vi "INIT_temp.vi"(8 "error in (no error)":errorcluster, 11 "DelayLineLS4 in":refnum<class "DelayLineLS4.lvclass">) -> (0 "error out":errorcluster, 3 "DelayLineLS4 out":refnum<class "DelayLineLS4.lvclass">)   [LabVIEW 2015, in "DelayLineLS4.lvclass"]
uses:
  DelayLineLS4.lvclass
  DelayLine.lvclass/DelayLine.ctl
  DelayLine.lvclass
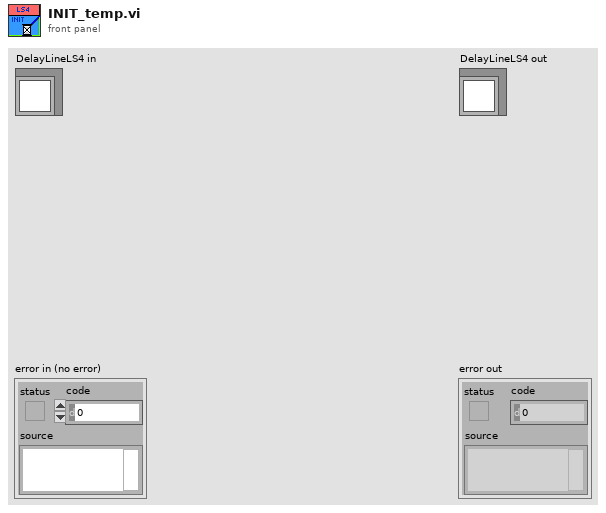
[diagram p1: front panel]
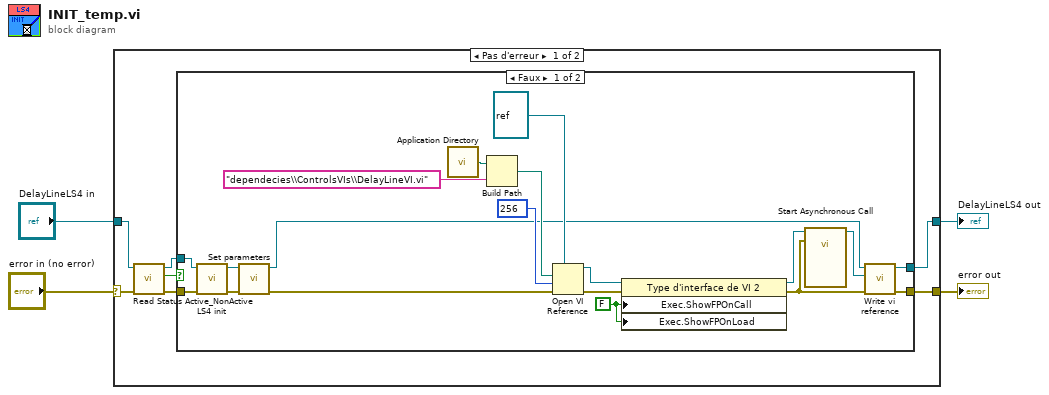
[diagram p0: block diagram]
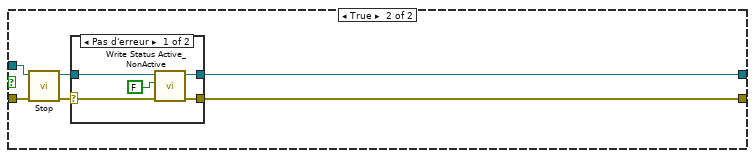
[diagram p2: hidden frame]
diagram:
  n1 = case shown="Pas d'erreur" "error in (no error)" {
    selector: "error in (no error)" -> [w8 w44]
    tunnel: "DelayLineLS4 in" -> [w7 w45]
    tunnel: [w6 w45] -> w1
    tunnel: [w5 w44] -> w2
    frame No Error {
      n2 = call "Read Status Active_NonActive.vi"("error in (no error)"=w8, "DelayLine in"=w7) -> ("error out"=w10:errorcluster, "Status Active/NonActive"=w9:bool, "DelayLine out"=w11:refnum<class "DelayLineLS4.lvclass">)  [unwired: 7 in]
      n3 = case shown="Faux" w9 {
        tunnel: w10 -> [w26 w33]
        tunnel: w11 -> [w27 w34]
        tunnel: [w30 w35] -> w5
        tunnel: [w29 w36] -> w6
        frame False {
          w15 = FALSE ("Execution:Show Front Panel On Call")
          n4 = call-dynamic "LS4 init.vi"("error in (no error)"=w26, "DelayLineLS4 in"=w27) -> ("error out"=w28:errorcluster, "DelayLineLS4 out"=w12:refnum<class "DelayLineLS4.lvclass">)  [unwired: 8 in]
          n5 = call-dynamic "Set parameters.vi"("error in (no error)"=w28, "DelayLineLS4 en entrée"=w12) -> ("error out"=w13:errorcluster, "DelayLineLS4 en sortie"=w17:refnum<class "DelayLineLS4.lvclass">)  [unwired: 8 in]
          n6 = call <vilib>:"Application Directory.vi"() -> ("Application Directory"=w23:path)
          n7 = Build Path(base path=w23, name or relative path="dependecies\\ControlsVIs\\DelayLineVI.vi") -> (appended path=w25:path)
          n8 = Open VI Reference(type specifier VI Refnum (for type only)=refnum<vi> refnum ("spécificateur de type du refnum de VI (pour type seulement)"), vi path=w25, options=256, error in (no error)=w13) -> (vi reference=w20:refnum<vi>, error out=w19:errorcluster)  [unwired: 2 in]
          n9 = property class="Type d'interface de VI 2"(reference=w20, error in=w19, "Exec.ShowFPOnCall"=w15, "Exec.ShowFPOnLoad"=w15) -> (reference out=w18:refnum<vi>, error out=w16:errorcluster)
          n10 = call-by-ref "Start Asynchronous Call"(reference=w18, error in=w16) -> (reference out=w14:refnum<vi>)  [unwired: 12 in, 1 out]
          n11 = call "Write vi reference.vi"("error in (no error)"=w16, "vi reference"=w14, "DelayLine in"=w17) -> ("error out"=w30:errorcluster, "DelayLine out"=w29:refnum<class "DelayLineLS4.lvclass">)  [unwired: 7 in]
        }
        frame True {
          n12 = call-dynamic "Stop.vi"("error in (no error)"=w33, "DelayLineLS4 in"=w34) -> ("error out"=w32:errorcluster, "DelayLineLS4 out"=w31:refnum<class "DelayLineLS4.lvclass">)  [unwired: 8 in]
          n13 = case shown="Pas d'erreur" w32 {
            selector: w32 -> [w39 w43]
            tunnel: w31 -> [w41 w42]
            tunnel: [w40 w42] -> w36
            tunnel: [w38 w43] -> w35
            frame No Error {
              n14 = call "Write Status Active_NonActive.vi"("error in (no error)"=w39, "Status Active/NonActive"=FALSE, "DelayLine in"=w41) -> ("error out"=w38:errorcluster, "DelayLine out"=w40:refnum<class "DelayLineLS4.lvclass">)  [unwired: 7 in]
            }
            frame Error {
            }
          }
        }
      }
    }
    frame Error {
    }
  }
  "error out" <- w2
  "DelayLineLS4 out" <- w1
